vi "TEST - Get Data TD from Datalog Ref.vi"(8 "error in (no error)":errorcluster) -> (0 "error out":errorcluster, 2 "pass":bool)   [LabVIEW 2020, in "test_openg_variant.lvlib"]
uses:
  test_openg_variant.lvlib
  source/library/openg_variant.lvlib
  <vilib>/addons/_JKI Toolkits/Caraya/classes/Test/Test.lvclass
  <vilib>/addons/_JKI Toolkits/Caraya/classes/Assert/Assert.lvclass
  <vilib>/addons/_JKI Toolkits/Caraya/classes/Assert/Assert True.vi
  source/library/Type Descriptor.ctl
panel:
  out "Test Name":string
  in  "Data Log File Refnum":refnum<k1>
  out "Failures":T2(array[cluster])
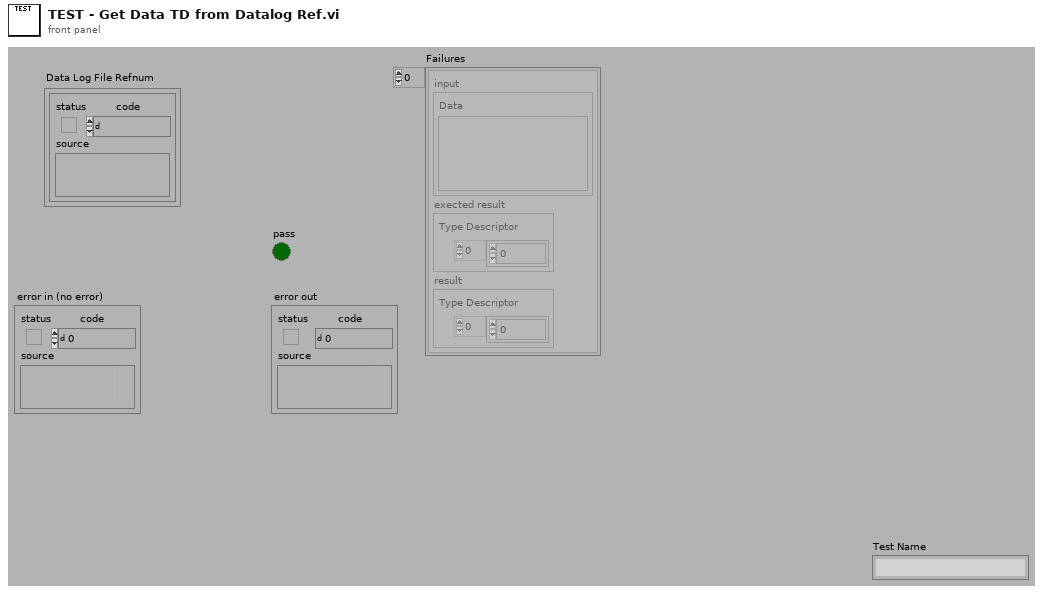
[diagram p1: front panel]
types:
  T1 = typedef "openg_variant.lvlib/Type Descriptor.ctl" = i16[]
  T2 = cluster{"input":cluster{"Data":variant}, "exected result":cluster{"Type Descriptor":T1}, "result":cluster{"Type Descriptor":T1}}[]
  T3 = cluster{"input":cluster{"Data":variant}, "exected result":cluster{"Type Descriptor":T1}, "result":cluster{"Type Descriptor":T1}}
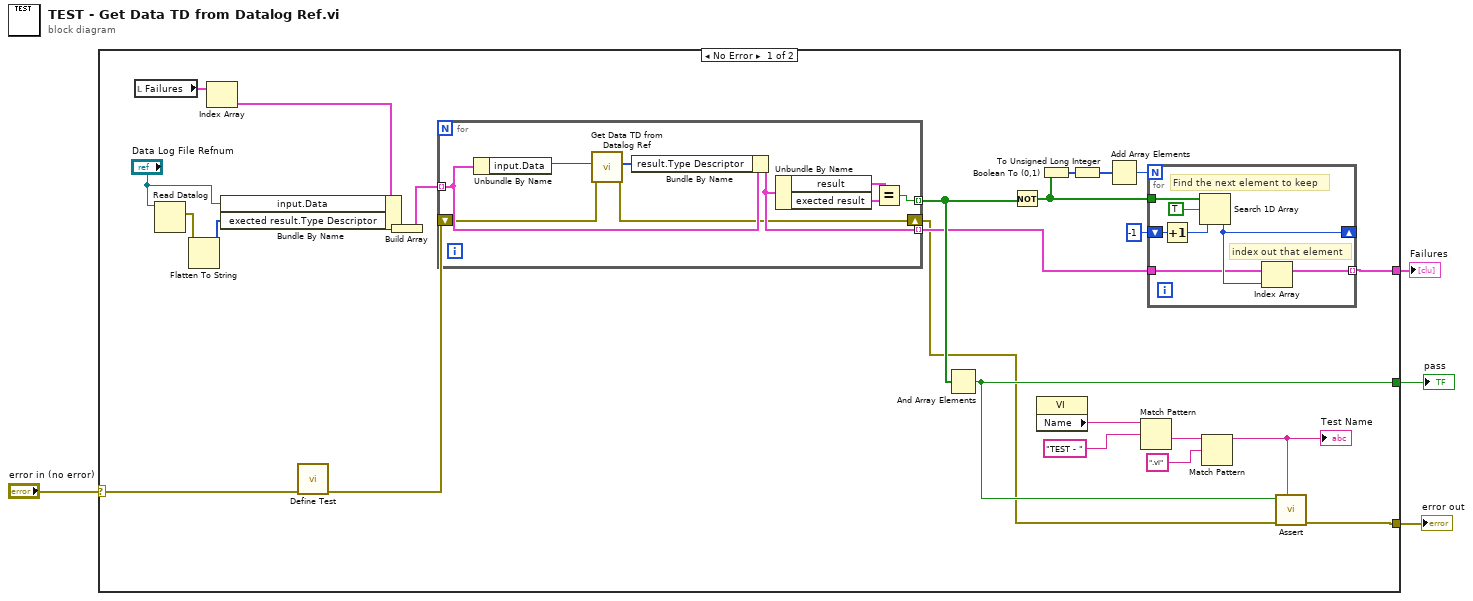
[diagram p0: block diagram]
diagram:
  n1 = case shown="No Error" "error in (no error)" {
    selector: "error in (no error)" -> [w7 w46]
    tunnel: [w8 _] -> w4
    tunnel: [w9 w46] -> w2
    tunnel: [w22 _] -> w1
    frame No Error {
      n2 = local read "Failures"() -> (w19:T2)
      n3 = Read Datalog(7:"Data Log File Refnum") -> (2:w17:errorcluster)  [unwired: 2 in, 2 out]
      n4 = Flatten To String(anything=w17) -> (type string=w16:i16[])  [unwired: 3 in, 2 out]
      n5 = Index Array(array=w19) -> (element=w18:T3)  [unwired: 1 in]
      n6 = Bundle By Name(cluster=w18, "input.Data"="Data Log File Refnum", "exected result.Type Descriptor"=w16) -> (w21:T3)
      n7 = call <vilib>:"Define Test.vi"("error in (no error)"=w7) -> ("error out"=w6:errorcluster)  [unwired: 9 in, 1 out]
      n8 = Build Array(w21) -> (w20:T2)
      n9 = for {
        tunnel: w20 -> [w44] mode=indexing
        tunnel: [w45] -> w24 mode=indexing
        tunnel: [w43] -> w23 mode=indexing
        shift-right: [w39] -> w5
        shift-left: w6 -> [w40]
        n10 = Unbundle By Name(w44) -> ("input.Data"=w37:variant)
        n11 = call "Get Data TD from Datalog Ref.vi"("error in (no error)"=w40, "Datalog Refnum"=w37) -> ("error out"=w39:errorcluster, "Type Descriptor"=w38:T1)  [unwired: 8 in]
        n12 = Bundle By Name(cluster=w44, "result.Type Descriptor"=w38) -> (w43:T3)
        n13 = Unbundle By Name(w43) -> ("result"=w42:cluster{"Type Descriptor":T1}, "exected result"=w41:cluster{"Type Descriptor":T1})
        n14 = Equal?(x=w42, y=w41) -> (x = y?=w45:bool)
      }
      n15 = And Array Elements(Boolean array=w24) -> (logical AND=w8:bool)
      n16 = Not(x=w24) -> (.not. x?=w26:bool[])
      n17 = property class="VI"() -> ("Name"=w13:string)  [unwired: 2 in, 2 out]
      n18 = Boolean To (0,1)(Boolean=w26) -> (0, 1=w27:i16[])
      n19 = To Unsigned Long Integer(number=w27) -> (unsigned 32bit integer=w25:u32[])
      n20 = Add Array Elements(numeric array=w25) -> (sum=w28:u32)
      n21 = Match Pattern(string=w13, regular expression="TEST - ") -> (after substring=w14:string)  [unwired: 1 in, 3 out]
      n22 = for {
        N: w28 -> [_]
        tunnel: w23 -> [w32]
        tunnel: w26 -> [w36]
        shift-right: [w33] -> _
        shift-left: -1 ("start index (0)") -> [w34]
        tunnel: [w31] -> w22 mode=indexing
        # "index out that element"
        # "Find the next element to keep"
        n23 = Increment(x=w34) -> (x+1=w30:i32)
        n24 = Search 1D Array(1D array=w36, element=TRUE, start index (0)=w30) -> (index of element=w33:i32)
        n25 = Index Array(array=w32, index=w33) -> (element=w31:T3)
      }
      n26 = Match Pattern(string=w14, regular expression=".vi") -> (before substring=w10:string)  [unwired: 1 in, 3 out]
      "Test Name" <- w10
      n27 = call-poly <vilib>:"Assert.vi"("Label"=w10, "error in (no error)"=w5, "True?"=w8) -> ("error out"=w9:errorcluster)  [unwired: 7 in, 1 out]
    }
    frame Error {
    }
  }
  "pass" <- w4
  "error out" <- w2
  "Failures" <- w1
